vi "Open.vi"(7 "Version":i32, 8 "error in (no error)":errorcluster caption="entrée d'erreur (pas d'erreur)", 11 "Path In":path) -> (0 "error out":errorcluster, 3 "Open Out":string)   [LabVIEW 2012, in "TiffLib.lvlib"]
uses:
  TiffLib.lvlib
  Librairies/TiffLib_v1/TiffLib_v1.lvlib
  Librairies/TiffLib_v2/TiffLib_v2.lvlib
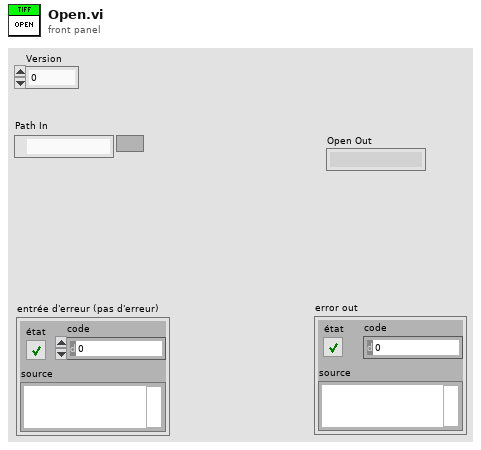
[diagram p1: front panel]
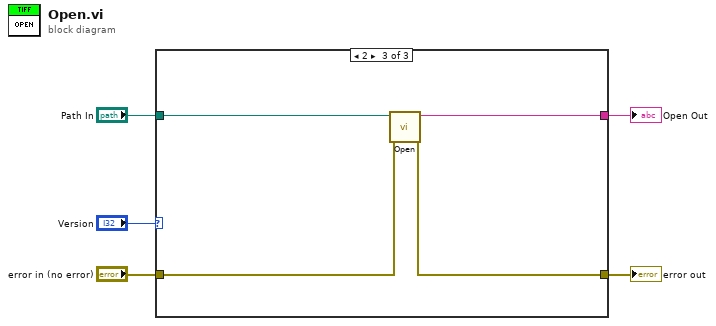
[diagram p0: block diagram]
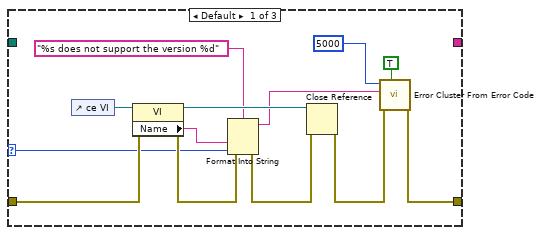
[diagram p2: hidden frame]
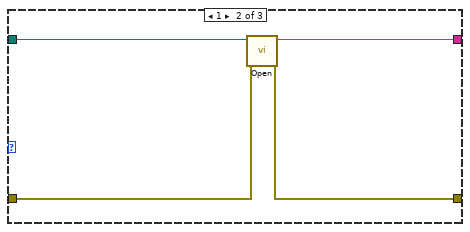
[diagram p3: hidden frame]
diagram:
  n1 = case shown="2" "Version" {
    selector: "Version" -> [w11 _ _]
    tunnel: "Path In" -> [_ w22 w26]
    tunnel: [_ w21 w25] -> w3
    tunnel: "error in (no error)" -> [w14 w20 w24]
    tunnel: [w18 w19 w23] -> w1
    frame Default {
      n2 = control-ref of="ce VI"() -> (w15:refnum<vi>)
      n3 = property class="VI"(reference=w15, error in=w14) -> (reference out=w10:refnum<vi>, error out=w13:errorcluster, "Name"=w12:string)
      n4 = Format Into String(format string="%s does not support the version %d" ("chaîne de format"), error in=w13, w12, w11) -> (resulting string=w7:string, error out=w9:errorcluster)  [unwired: 1 in]
      n5 = Close Reference(reference=w10, error in (no error)=w9) -> (error out=w8:errorcluster)
      n6 = call <vilib>:"Error Cluster From Error Code.vi"("show call chain? (False)"=TRUE, "error in (no error)"=w8, "error message (\"\")"=w7, "error code (0)"=5000) -> ("error out"=w18:errorcluster)  [unwired: 5 in]
    }
    frame 1 {
      n7 = call "Open.vi"("error in (no error)"=w20, "Path In"=w22) -> ("error out"=w19:errorcluster, "Open Out"=w21:string)  [unwired: 8 in]
    }
    frame 2 {
      n8 = call "Open.vi"("error in (no error)"=w24, "Path In"=w26) -> ("error out"=w23:errorcluster, "Open Out"=w25:string)  [unwired: 8 in]
    }
  }
  "Open Out" <- w3
  "error out" <- w1
